vi "Get Instrument Version.vi"(8 "error in":errorcluster, 11 "Instruments in":refnum<class "Instruments.lvclass">) -> (0 "error out":errorcluster, 1 "Version":string, 2 "Driver":string, 3 "Instruments out":refnum<class "Instruments.lvclass">)   [LabVIEW 2023, in "Instruments.lvlib" / "Instruments.lvclass"]
uses:
  Library/Instruments.lvclass
  <vilib>/Utility/LVLibp/NI_PackedLibraryUtility.lvlib
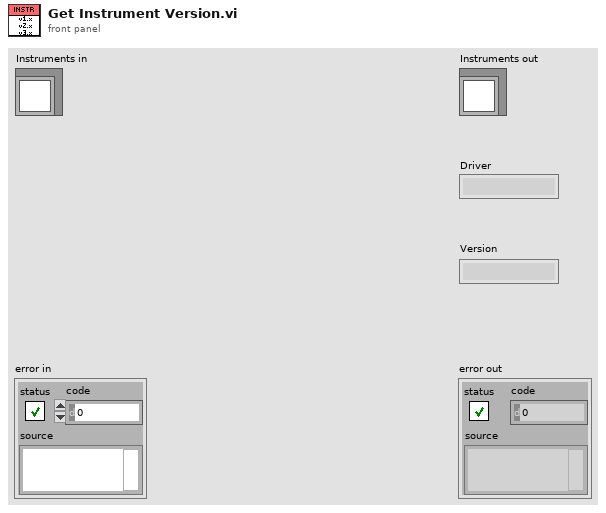
[diagram p1: front panel]
types:
  T1 = cluster{"Major":u16, "Minor":u16, "Fix":u16, "Build":u16}
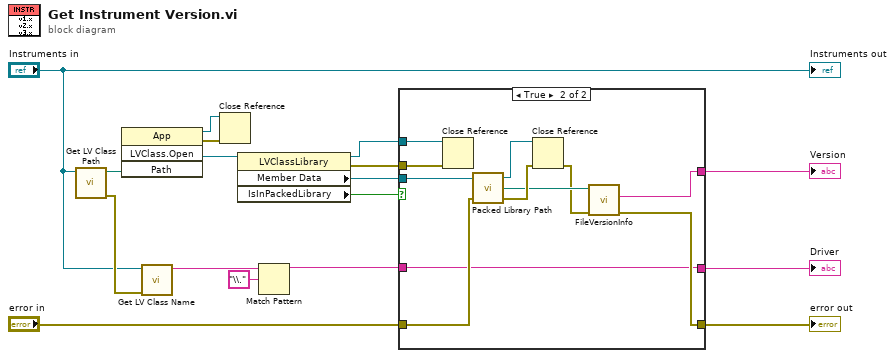
[diagram p0: block diagram]
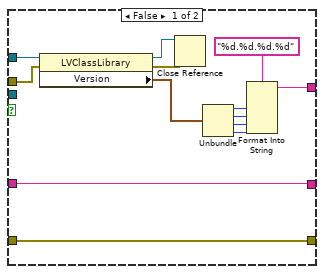
[diagram p2: hidden frame]
diagram:
  n1 = call <vilib>:"Get LV Class Path.vi"("object"="Instruments in") -> ("error out"=w6:errorcluster, "class path"=w14:path)  [unwired: 9 in]
  n2 = invoke class="App" method="LVClass.Open"("Path"=w14) -> (reference out=w13:refnum<vi>, error out=w12:errorcluster, "LVClass.Open"=w10:refnum<vi>)  [unwired: 3 in, 1 out]
  n3 = call <vilib>:"Get LV Class Name.vi"("error in (no error)"=w6, "object"="Instruments in") -> ("class name"=w3:string)  [unwired: 8 in, 1 out]
  n4 = Close Reference(reference=w13, error in (no error)=w12) -> ()  [unwired: 1 out]
  n5 = property class="LVClassLibrary"(reference=w10) -> (reference out=w17:refnum<vi>, error out=w16:errorcluster, "Member Data"=w11:refnum<vi>, "IsInPackedLibrary"=w15:bool)  [unwired: 1 in]
  n6 = Match Pattern(string=w3, regular expression="\\.") -> (before substring=w2:string)  [unwired: 1 in, 3 out]
  n7 = case shown="True" w15 {
    tunnel: w11 -> [_ w41]
    tunnel: [w21 w40] -> w7
    tunnel: "error in" -> [w19 w32]
    tunnel: w16 -> [w29 w36]
    tunnel: w17 -> [w30 w35]
    tunnel: [w19 w34] -> w8
    tunnel: w2 -> [w18 w31]
    tunnel: [w18 w31] -> w1
    frame False {
      n8 = property class="LVClassLibrary"(reference=w30, error in=w29) -> (reference out=w27:refnum<vi>, error out=w28:errorcluster, "Version"=w26:T1)
      n9 = Close Reference(reference=w27, error in (no error)=w28) -> ()  [unwired: 1 out]
      n10 = Unbundle(w26) -> ("Major"=w25:u16, "Minor"=w24:u16, "Fix"=w23:u16, "Build"=w22:u16)
      n11 = Format Into String(format string="%d.%d.%d.%d", w25, w24, w23, w22) -> (resulting string=w21:string)  [unwired: 2 in, 1 out]
    }
    frame True {
      n12 = Close Reference(reference=w35, error in (no error)=w36) -> ()  [unwired: 1 out]
      n13 = call <vilib>:"Packed Library Path.vi"("error in (no error)"=w32, "vi reference"=w41) -> ("error out"=w38:errorcluster, "packed library path"=w37:path, "vi reference out"=w39:refnum<vi>)  [unwired: 1 in]
      n14 = Close Reference(reference=w39, error in (no error)=w38) -> (error out=w33:errorcluster)
      n15 = call <vilib>:"FileVersionInfo.vi"("error in (no error)"=w33, "Application Path in"=w37) -> ("error out"=w34:errorcluster, "File Version Info"=w40:string)  [unwired: 6 in, 2 out]
    }
  }
  "error out" <- w8
  "Version" <- w7
  "Driver" <- w1
  "Instruments out" <- "Instruments in"
